vi "Make.vi"(8 "error in (no error)":errorcluster, 9 "Item Refnum":refnum<vi>, 10 "Target":refnum<vi>, 11 "Concrete Message Rescripter":refnum<class "Concrete Message Rescripter.lvclass">) -> (0 "error out":errorcluster, 3 "Concrete Message Rescripter out":refnum<class "Concrete Message Rescripter.lvclass">)   [LabVIEW 2020, in "Message Rescripter.lvlib" / "Concrete Message Rescripter.lvclass"]
uses:
  Concrete Message Rescripter.lvclass
  MessageMakerProvider/_Message Maker/_Maker Classes/Message Scripter/Message Scripter.lvclass
  Message Rescripter.lvlib
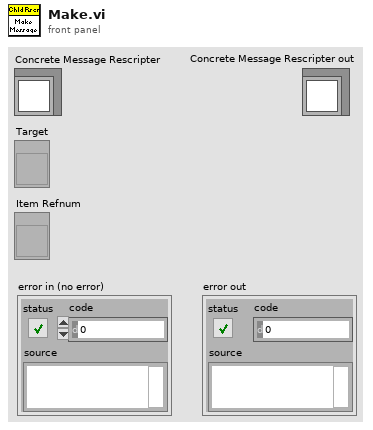
[diagram p1: front panel]
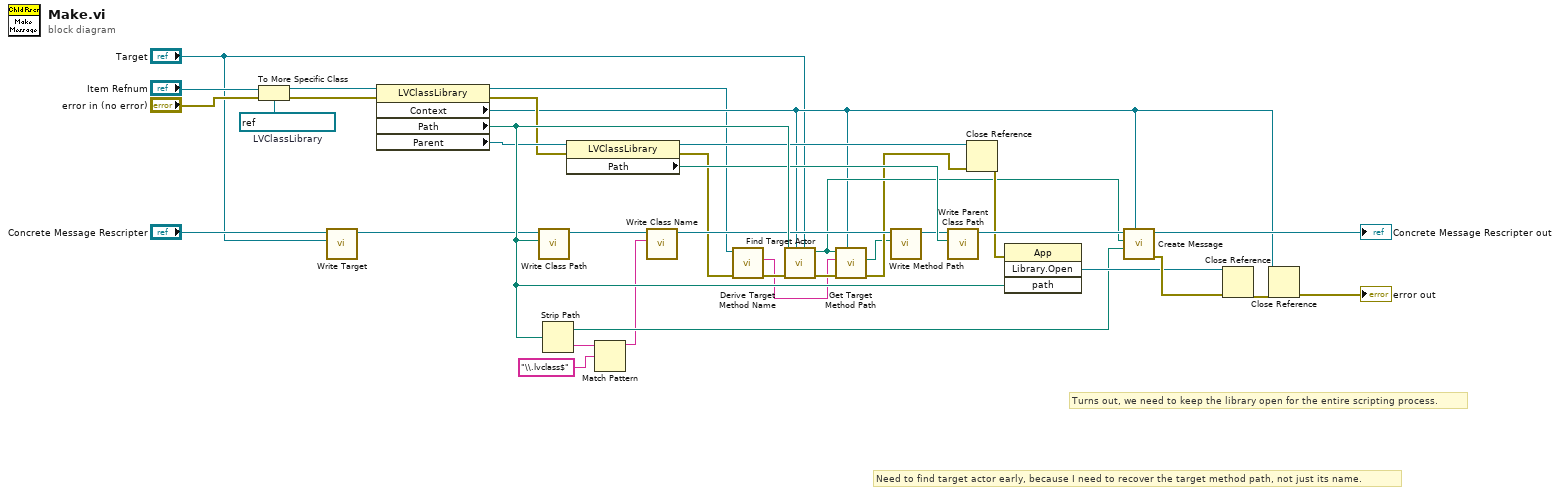
[diagram p0: block diagram]
diagram:
  w35 = refnum<vi> refnum  # LVClassLibrary
  # "Need to find target actor early, because I need to recover the target method path, not just its name."
  # "Turns out, we need to keep the library open for the entire scripting process."
  n1 = To More Specific Class(target class=w35, reference="Item Refnum", error in="error in (no error)") -> (specific class reference=w33:refnum<vi>, error out=w34:errorcluster)
  n2 = call "Write Target.vi"("Target"="Target", "Message Scripter in"="Concrete Message Rescripter") -> ("Message Scripter out"=w4:refnum<class "Concrete Message Rescripter.lvclass">)  [unwired: 9 in]
  n3 = property class="LVClassLibrary"(reference=w33, error in=w34) -> (reference out=w8:refnum<vi>, error out=w22:errorcluster, "Context"=w12:refnum<vi>, "Path"=w36:path, "Parent"=w23:refnum<vi>)
  n4 = call "Write Class Path.vi"("Class Path"=w36, "Message Scripter in"=w4) -> ("Message Scripter out"=w28:refnum<class "Concrete Message Rescripter.lvclass">)  [unwired: 9 in]
  n5 = Strip Path(path=w36) -> (stripped path=w29:path, name=w11:string)
  n6 = property class="LVClassLibrary"(reference=w23, error in=w22) -> (reference out=w18:refnum<vi>, error out=w6:errorcluster, "Path"=w20:path)
  n7 = Match Pattern(string=w11, regular expression="\\.lvclass$") -> (before substring=w10:string)  [unwired: 1 in, 3 out]
  n8 = call "Write Class Name.vi"("Class Name"=w10, "Message Scripter in"=w28) -> ("Message Scripter out"=w17:refnum<class "Concrete Message Rescripter.lvclass">)  [unwired: 9 in]
  n9 = call "Derive Target Method Name.vi"("error in (no error)"=w6, "Library"=w8) -> ("error out"=w9:errorcluster, "Likely Target Method"=w3:string)  [unwired: 8 in]
  n10 = call "Find Target Actor.vi"("Target"="Target", "App Inst"=w12, "error in (no error)"=w9, "Message Path"=w36) -> ("error out"=w16:errorcluster, "Targeted Actor"=w14:path)  [unwired: 6 in]
  n11 = call "Get Target Method Path.vi"("App Inst"=w12, "error in (no error)"=w16, "Target Method"=w3, "Target Actor Path"=w14) -> ("error out"=w13:errorcluster, "Target Method Path"=w2:path)  [unwired: 6 in]
  n12 = call "Write Method Path.vi"("Method Path"=w2, "Message Scripter in"=w17) -> ("Message Scripter out"=w15:refnum<class "Concrete Message Rescripter.lvclass">)  [unwired: 9 in]
  n13 = call-dynamic "Write Parent Class Path.vi"("Parent Class Path"=w20, "Concrete Message Scripter in"=w15) -> ("Concrete Message Scripter out"=w21:refnum<class "Concrete Message Rescripter.lvclass">)  [unwired: 9 in]
  n14 = Close Reference(reference=w18, error in (no error)=w13) -> (error out=w19:errorcluster)
  n15 = invoke class="App" method="Library.Open"(error in=w19, "path"=w36) -> ("Open Library"=w30:refnum<vi>)  [unwired: 2 in, 3 out]
  n16 = call "Create Message.vi"("AppInst"=w12, "Destination Path"=w29, "Actor class path"=w14, "Message Maker in"=w21) -> ("error out"=w31:errorcluster, "Message Maker out"=→"Concrete Message Rescripter out":refnum<class "Concrete Message Rescripter.lvclass">)  [unwired: 6 in]
  n17 = Close Reference(reference=w30, error in (no error)=w31) -> (error out=w32:errorcluster)
  n18 = Close Reference(reference=w12, error in (no error)=w32) -> (error out=→"error out":errorcluster)
